vi "MTool34450A.vi"(6 "error in (no error)":errorcluster, 8 "Ringfor34450A":u16(ring) items=["SYSTem:VERSion?", "SYSTem:ERRor?", "*IDN?", "MEAS:CURR:DC?", "MEAS:VOLT?", "SYSTem:ERRor?", ""], 9 "RingforIT8511":u16(ring) items=["SYSTem:VERSion?", "SYSTem:ERRor?", "*IDN?", "MEAS:CURR:DC?", "MEAS:VOLT?", "MEAS:VOLT:DC?"], 10 "VISA resource name":refnum<visa-resource-name>="USB0::0x2A8D::0xB318::MY59430005::INSTR", 11 "ChangeStatus":u16(ring) items=["IT8511", "34450A", "WRBuff"]) -> (0 "error out":errorcluster, 1 "μA":string, 2 "μA":dbl format="%#_6f", 3 "read buffer":string)   [LabVIEW 2019]
panel:
  out "Numeric":dbl
  out "hex integer string":string
  in  "Boolean 2":bool
  in  "milliseconds to wait":u32
  in  "write buffer":string
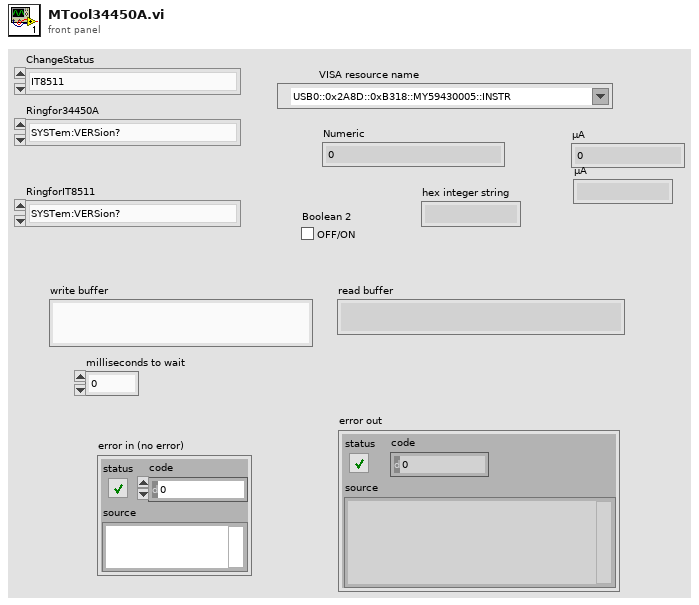
[diagram p1: front panel]
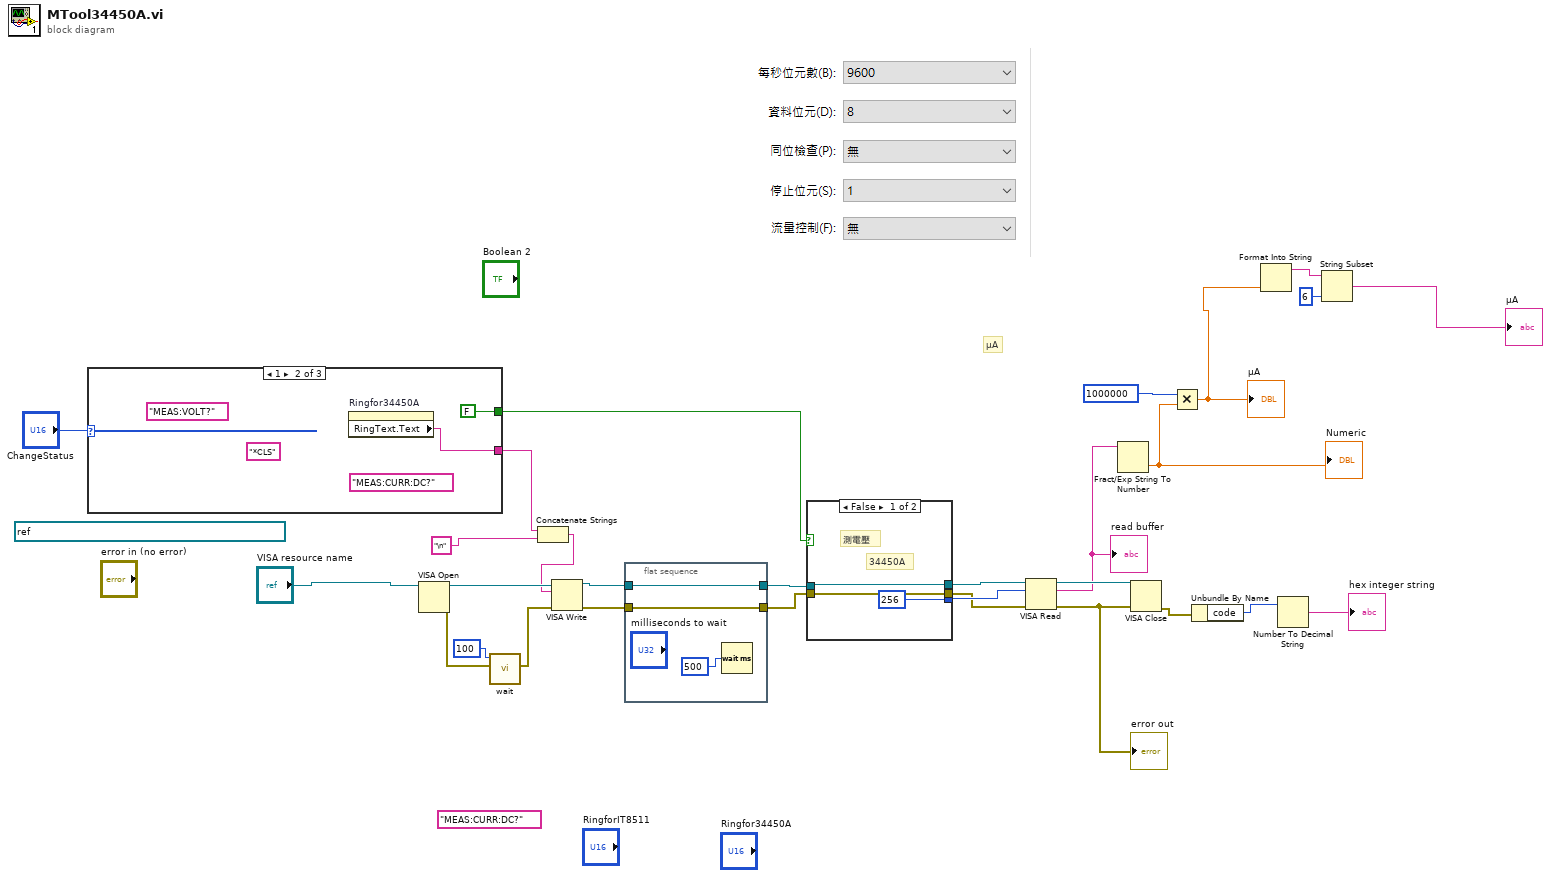
[diagram p0: block diagram]
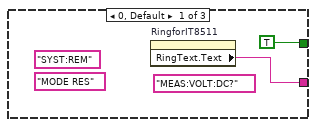
[diagram p2: hidden frame]
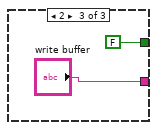
[diagram p3: hidden frame]
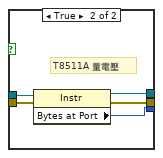
[diagram p4: hidden frame]
diagram:
  (unwired) "MEAS:CURR:DC?" ("string")
  (unwired) refnum<visa-resource-name> "USB0::0x2A8D::0xB318::MY59430005::INSTR" ("VISA resource name")
  # "μA"
  n1 = case shown="1" "ChangeStatus" {
    tunnel: [w30 w32 "write buffer"] -> w15
    tunnel: [TRUE FALSE FALSE] -> w14
    frame 0, Default {
      (unwired) "MODE RES" ("string")
      (unwired) "SYST:REM" ("string")
      (unwired) "MEAS:VOLT:DC?" ("string")
      n2 = property on="RingforIT8511" class="Ring (strict)"() -> ("RingText.Text"=w30:string)  [unwired: 2 in, 2 out]
    }
    frame 1 {
      (unwired) "*CLS" ("string")
      (unwired) "MEAS:CURR:DC?" ("string")
      (unwired) "MEAS:VOLT?" ("string")
      n3 = property on="Ringfor34450A" class="Ring (strict)"() -> ("RingText.Text"=w32:string)  [unwired: 2 in, 2 out]
    }
    frame 2 {
    }
  }
  n4 = VISA Open(VISA resource name="VISA resource name") -> (VISA resource name=w29:refnum<visa-resource-name>, error out=w8:errorcluster)  [unwired: 4 in]
  n5 = call "wait.vi"("error in"=w8, "wait(ms)"=100) -> ("error out"=w7:errorcluster)  [unwired: 9 in]
  n6 = Concatenate Strings(w15, "\n" ("string")) -> (w20:string)
  n7 = VISA Write(VISA resource name=w29, write buffer=w20, error in (no error)=w7) -> (VISA resource name out=w24:refnum<visa-resource-name>, error out=w27:errorcluster)  [unwired: 1 out]
  n8 = flat-sequence {
    tunnel: w27 -> [w38]
    tunnel: [w38] -> w23
    tunnel: [w37] -> w25
    tunnel: w24 -> [w37]
    frame #0 {
      n9 = Wait (ms)(milliseconds to wait=500) -> ()  [unwired: 1 out]
    }
  }
  n10 = case shown="False" w14 {
    tunnel: [u32 256 ("Bytes at Port") w46] -> w26
    tunnel: w25 -> [w41 w45]
    tunnel: w23 -> [w40 w44]
    tunnel: [w40 w43] -> w22
    tunnel: [w41 w42] -> w21
    frame False {
      # "測電壓"
      # "34450A"
    }
    frame True {
      # "T8511A 量電壓"
      n11 = property class="Instr"(reference=w45, error in=w44) -> (reference out=w42:refnum<visa-resource-name>, error out=w43:errorcluster, "Bytes at Port"=w46:u32)
    }
  }
  n12 = VISA Read(VISA resource name=w21, byte count=w26, error in (no error)=w22) -> (VISA resource name out=w28:refnum<visa-resource-name>, read buffer=w12:string, error out=w16:errorcluster)  [unwired: 1 out]
  "read buffer" <- w12
  "error out" <- w16
  n13 = Fract/Exp String To Number(string=w12) -> (number=w10:dbl)  [unwired: 3 in, 1 out]
  "Numeric" <- w10
  n14 = VISA Close(VISA resource name=w28, error in (no error)=w16) -> (error out=w17:errorcluster)
  n15 = Multiply(x=1000000, y=w10) -> (x*y=w2:dbl)
  "μA" <- w2
  n16 = Unbundle By Name(w17) -> ("code"=w19:i32)
  n17 = Format Into String(w2) -> (resulting string=w3:string)  [unwired: 3 in, 1 out]
  n18 = Number To Decimal String(number=w19) -> (decimal integer string=→"hex integer string":string)  [unwired: 1 in]
  n19 = String Subset(string=w3, length (rest)=6 ("length (rest)")) -> (substring=→"μA":string)  [unwired: 1 in]
